vi "Panel.vi"(11 "Team Field Panel in":refnum<class "Team Field Panel.lvclass">) -> ()   [LabVIEW 2020, in "SB App.lvlib" / "Team Field Panel.lvclass"]
uses:
  Team Field Panel.lvclass
  C:/Program Files (x86)/National Instruments/LabVIEW 2020/vi.lib/IlluminatedG/IG OOPanel/OOPanel/Panel/Panel.lvclass
  <vilib>/IlluminatedG/IG OOPanel/OOPanel/Panel/Basic UI State.ctl
  Team Field Panel.lvclass/Team Field Panel.ctl
  <vilib>/IlluminatedG/IG OOPanel/OOPanel/Panel/Panel.lvclass
  <vilib>/IlluminatedG/IG OOPanel/OOPanel/OOPanel.lvlib
  SquareBattle/SquareBattle.lvlib
panel:
  out "Team Field":i32[][](graph)
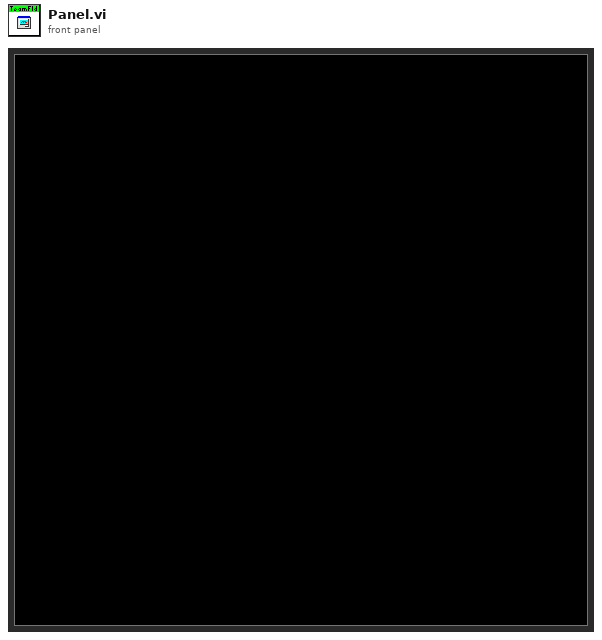
[diagram p1: front panel]
types:
  T1 = typedef "OOPanel.lvlib/Panel.lvclass/Basic UI State.ctl" = enum16{"Init", "Run", "Close"}
  T2 = typedef "SB App.lvlib/Team Field Panel.lvclass/Incoming Events.ctl" = cluster{"Team Map Update":refnum<user-event>}
  T3 = typedef "OOPanel.lvlib/Panel.lvclass/Panel Events.ctl" = cluster{"Visbility":refnum<user-event>, "Close":refnum<user-event>}
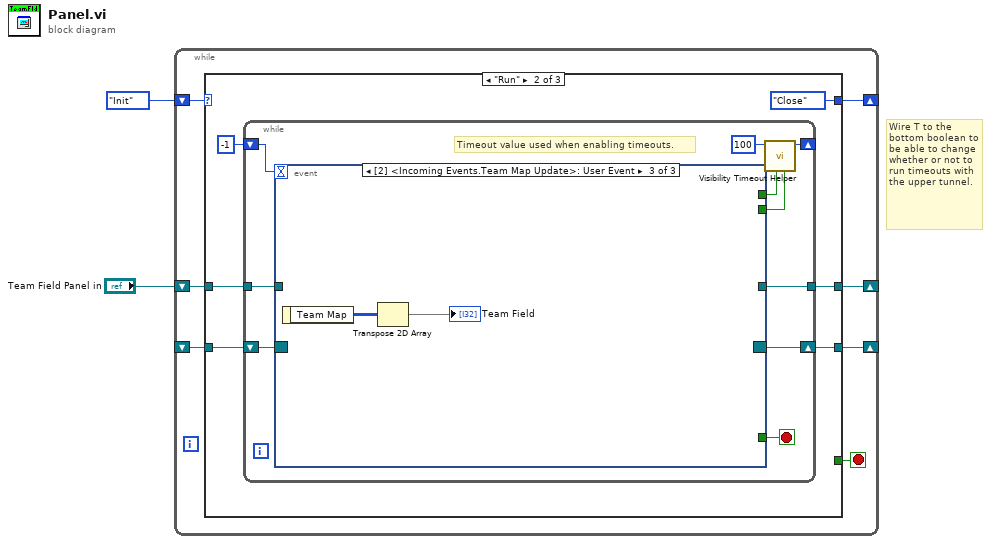
[diagram p0: block diagram]
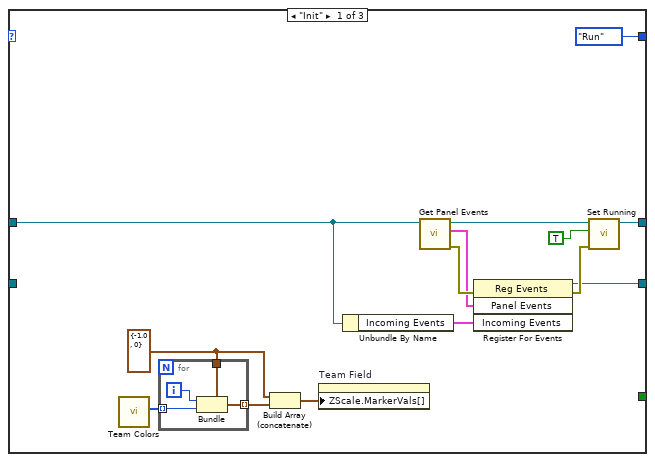
[diagram p2: hidden frame]
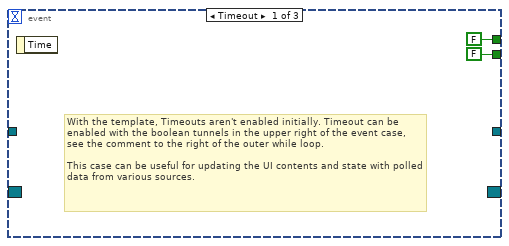
[diagram p3: hidden frame]
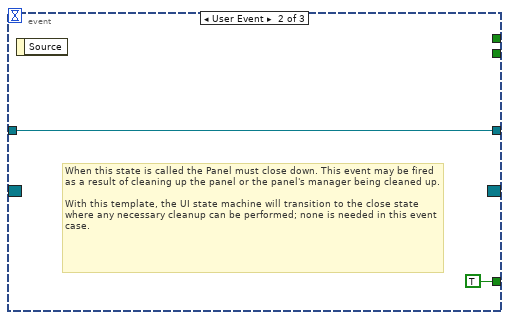
[diagram p4: hidden frame]
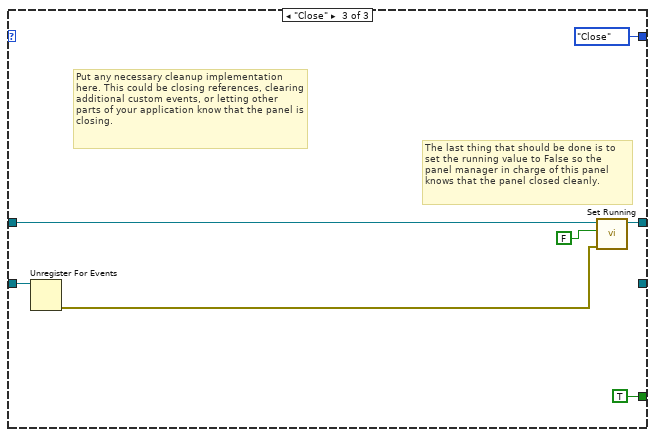
[diagram p5: hidden frame]
diagram:
  # "Wire T to the bottom boolean to be able to change whether or not to run timeouts with the upper tunnel."
  n1 = while {
    shift-right: [w8] -> _
    shift-left: _ -> [w9]
    shift-right: [w6] -> _
    shift-left: Basic_UI_State."Init" ("Basic UI State") -> [w7]
    shift-right: [w4] -> _
    shift-left: "Team Field Panel in" -> [w3]
    stop <- w5 stop-if-true
    n2 = case shown="\"Run\"" w7 {
      tunnel: w9 -> [_ w33 w52]
      tunnel: [w17 w31 _] -> w8
      tunnel: [Basic_UI_State."Run" ("Basic UI State") Basic_UI_State."Close" ("Basic UI State") Basic_UI_State."Close" ("Basic UI State")] -> w6
      tunnel: [_ _ TRUE] -> w5
      tunnel: [w16 w28 w50] -> w4
      tunnel: w3 -> [w14 w29 w51]
      frame "Init" {
        w11 = cluster{dbl, u32} {-1.0, 0}
        n3 = call "Team Colors.vi"() -> ("Team Colors"=w15:u32[])  [unwired: 11 in]
        n4 = for {
          tunnel: w15 -> [w27] mode=indexing
          tunnel: w11 -> [w26]
          tunnel: [w24] -> w12 mode=indexing
          i -> [w25]
          n5 = Bundle(cluster=w26, w25, w27) -> (w24:cluster{dbl, u32})
        }
        n6 = Build Array (concatenate)(w11, w12) -> (w10:cluster{dbl, u32}[])
        n7 = property on="Team Field" class="IntGraph (strict)"("ZScale.MarkerVals[]"=w10) -> ()  [unwired: 2 in, 2 out]
        n8 = Unbundle By Name(w14) -> ("Incoming Events"=w13:T2)
        n9 = call <vilib>:"Get Panel Events.vi"("Panel in"=w14) -> ("error out"=w23:errorcluster, "Panel Events"=w19:T3, "Panel out"=w20:refnum<class "Team Field Panel.lvclass">)  [unwired: 8 in]
        n10 = register-events(error in=w23, w19, w13) -> (reference out=w17:refnum<event-registration>, error out=w21:errorcluster)  [unwired: 1 in]
        n11 = call <vilib>:"Set Running.vi"("error in (no error)"=w21, "Running"=TRUE, "Panel in"=w20) -> ("Panel out"=w16:refnum<class "Team Field Panel.lvclass">)  [unwired: 7 in, 1 out]
      }
      frame "Run" {
        n12 = while {
          shift-right: [w39] -> w31
          shift-left: w33 -> [w40]
          shift-right: [w42] -> _
          shift-left: -1 ("Timeout") -> [w41]
          tunnel: w29 -> [w35]
          tunnel: [w34] -> w28
          stop <- w36 stop-if-true
          # "Timeout value used when enabling timeouts."
          n13 = event shown="[2] <Incoming Events.Team Map Update>: User Event" {
            selector: w40 -> [_ _ _]
            dyn-events: [_ _ _] -> w39
            timeout: w41 -> [_ _ _]
            tunnel: [FALSE _ _] -> w38
            tunnel: [FALSE _ _] -> w37
            tunnel: [_ TRUE _] -> w36
            tunnel: w35 -> [_ w46 _]
            tunnel: [_ w46 _] -> w34
            event Timeout {
              # "With the template, Timeouts aren't enabled initially. Timeout can be enabled with the boolean tunnels in the upper right of the event case, see the comment to the right of the outer while loop.\n\nThis case can be useful for updating the UI contents and state with polled data from various sources."
              n14 = event-data() -> ()  [unwired: 1 in, 1 out]
            }
            event User Event {
              # "When this state is called the Panel must close down. This event may be fired as a result of cleaning up the panel or the panel's manager being cleaned up.\n\nWith this template, the UI state machine will transition to the close state where any necessary cleanup can be performed; none is needed in this event case."
              n15 = event-data() -> ()  [unwired: 1 in, 1 out]
            }
            event User Event {
              n16 = event-data() -> ("Team Map"=w49:i32[][])  [unwired: 1 in]
              n17 = Transpose 2D Array(2D array=w49) -> (transposed array=→"Team Field":i32[][])
            }
          }
          n18 = call <vilib>:"Visibility Timeout Helper.vi"("Update?"=w37, "Use Timeout?"=w38, "Visible Timeout mS"=100) -> ("Timeout"=w42:i32)  [unwired: 8 in]
        }
      }
      frame "Close" {
        # "Put any necessary cleanup implementation here. This could be closing references, clearing additional custom events, or letting other parts of your application know that the panel is closing."
        # "The last thing that should be done is to set the running value to False so the panel manager in charge of this panel knows that the panel closed cleanly."
        n19 = Unregister For Events(event registration refnum=w52) -> (error out=w54:errorcluster)  [unwired: 1 in]
        n20 = call <vilib>:"Set Running.vi"("error in (no error)"=w54, "Running"=FALSE, "Panel in"=w51) -> ("Panel out"=w50:refnum<class "Team Field Panel.lvclass">)  [unwired: 7 in, 1 out]
      }
    }
  }
